vi "Initiate Sampling.vi"(7 "display string (none)":string, 8 "error in":errorcluster, 9 "stream mode (False)":bool, 10 "ARM mode (SGL)":T1=enum."SGL", 11 "VISA resource in":refnum<visa-resource-name>) -> (0 "error out":errorcluster, 3 "VISA resource out":refnum<visa-resource-name>)   [LabVIEW 2013, in "3458A Virtual Digitizer.lvlib" / "3458A Digitizing Low Levels.lvlib"]
doc: "Arms DMM so it may start digitizing depending on the mode setting. \n\nNote: Reentrant VI so it can be executed in parallel for multiple 3458A sessions."
uses:
  3458A Digitizing Low Levels.lvlib
  Configure/First Sample Trigger.ctl
  3458A Basic Driver/3458A Basic Driver.lvlib
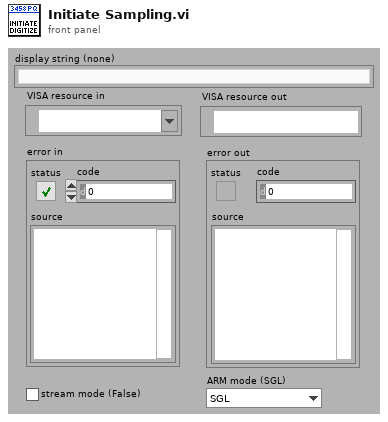
[diagram p1: front panel]
types:
  T1 = typedef "3458A Virtual Digitizer.lvlib/3458A Digitizing Low Levels.lvlib/First Sample Trigger.ctl" = enum16{"AUTO", "EXT", "SYN", "SGL", "HOLD", "LEVEL"}
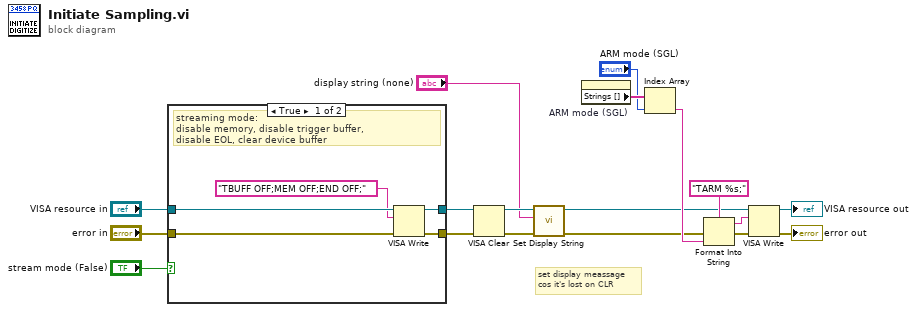
[diagram p0: block diagram]
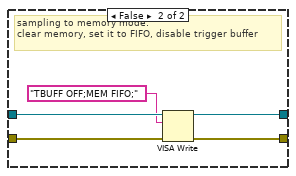
[diagram p2: hidden frame]
diagram:
  # "set display meassage\ncos it's lost on CLR"
  n1 = case shown="True" "stream mode (False)" {
    tunnel: "error in" -> [w23 w28]
    tunnel: "VISA resource in" -> [w22 w27]
    tunnel: [w19 w24] -> w6
    tunnel: [w20 w25] -> w7
    frame True {
      # "streaming mode:\ndisable memory, disable trigger buffer,\ndisable EOL, clear device buffer"
      n2 = VISA Write(VISA resource name=w22, write buffer="TBUFF OFF;MEM OFF;END OFF;", error in (no error)=w23) -> (VISA resource name out=w19:refnum<visa-resource-name>, error out=w20:errorcluster)  [unwired: 1 out]
    }
    frame False {
      # "sampling to memory mode:\nclear memory, set it to FIFO, disable trigger buffer"
      n3 = VISA Write(VISA resource name=w27, write buffer="TBUFF OFF;MEM FIFO;", error in (no error)=w28) -> (VISA resource name out=w24:refnum<visa-resource-name>, error out=w25:errorcluster)  [unwired: 1 out]
    }
  }
  n4 = VISA Clear(VISA resource name=w6, error in (no error)=w7) -> (VISA resource name out=w4:refnum<visa-resource-name>, error out=w5:errorcluster)
  n5 = call "Set Display String.vi"("error in(no error)"=w5, "display string (none)"="display string (none)", "VISA Resource Name"=w4) -> ("error out"=w3:errorcluster, "VISA resource name out"=w2:refnum<visa-resource-name>)  [unwired: 7 in]
  n6 = property on="ARM mode (SGL)" class="Enum (strict)"() -> ("Strings []"=w14:string[])  [unwired: 2 in, 2 out]
  n7 = Index Array(array=w14, index="ARM mode (SGL)") -> (element=w9:string)
  n8 = Format Into String(format string="TARM %s;" ("write buffer"), error in=w3, w9) -> (resulting string=w10:string, error out=w12:errorcluster)  [unwired: 1 in]
  n9 = VISA Write(VISA resource name=w2, write buffer=w10, error in (no error)=w12) -> (VISA resource name out=→"VISA resource out":refnum<visa-resource-name>, error out=→"error out":errorcluster)  [unwired: 1 out]
